vi "JSON Config Update Test Cases.vi"() -> ()   [LabVIEW 2021]
uses:
  CIFUtilities/CIFOutOfBand/CIFOutOfBand.lvclass/CIFOutOfBand.ctl
  CIFTemplateCoreOOB/OOB_Rx/Private/Command Settings.vi
  CIFUtilities/CIFOutOfBand/Accessors/Write Local OOB Data.vi
  CIFUtilities/CIFOutOfBand/Accessors/Read Local OOB Data.vi
  CIFUtilities/CIFOutOfBand/Read OOB DVR.vi
  CIFTemplateCoreOOB/OOB_Rx/Private/Read Payload.vi
  CIFUtilities/CIFOutOfBand/Write OOB DVR.vi
  CIFUtilities/CIFOutOfBand/Utilities/Command to Bitwise Command.vi
  CIFTemplateCoreOOB/OOB_Rx/CIFTemplateCoreOOB_Rx.lvclass
  D:/dev/CIF-Core-LabVIEW/src/CIFUtilities/CIFOutOfBand/CIFOutOfBand.lvclass
  CIFUtilities/CIFOutOfBand/Init OOB.vi
  <vilib>/addons/_JKI.lib/Serialization/JSON/Library/Unflatten From JSON String.vi
  <vilib>/addons/_JKI.lib/Serialization/JSON/JKI JSON Serialization.lvlib
  CIFUtilities/CIFOutOfBand/CIFOutOfBand.lvclass
panel:
  out "pass":bool
  out "error out":errorcluster
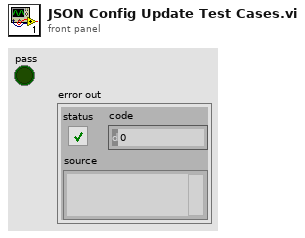
[diagram p1: front panel]
types:
  T1 = cluster{"Numeric":dbl, "String":string, "Boolean":bool}[]
  T2 = cluster{"Numeric":dbl, "Array":cluster{"Numeric":dbl, "String":string, "Boolean":bool}[], "string":string, "Null array":u8[]}
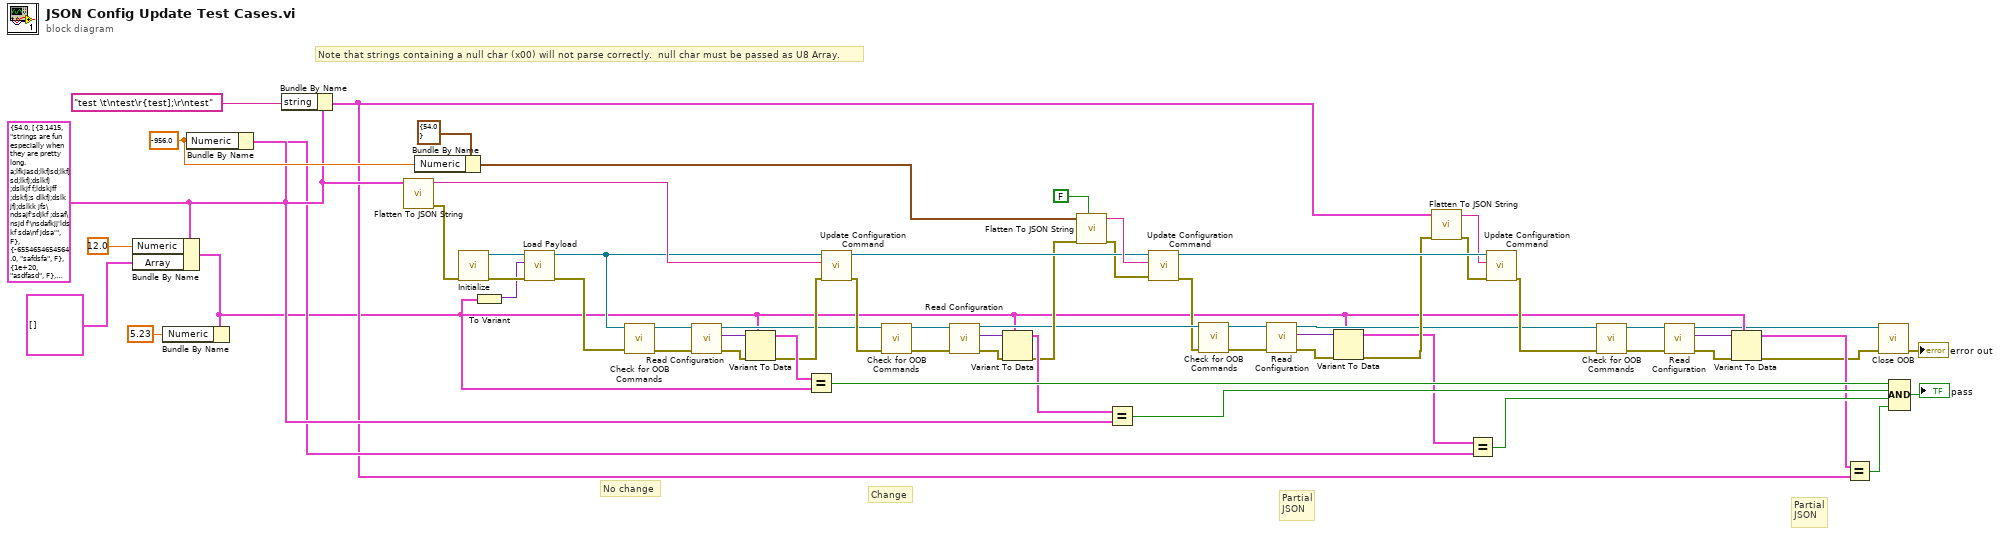
[diagram p0: block diagram]
diagram:
  w53 = -956.0 ("Numeric")
  w46 = T2 {"Numeric"=54.0, "Array"=[{"Numeric"=3.1415, "String"="strings are fun especially when they are pretty long. a;lfkjasd;lkfjsd;lkfjsd;lkfj;dslkfj ;dslkjf f;ldskjff ;dskfj;s dlkfj;dslk jfj;dslkk jfs\ndsajf'sdjkf ;dsaf\nsjd f'\nsdafkjj'lds kf sda\nf jdsa'", "Boolean"=FALSE}, {"Numeric"=-6554654654564.0, "String"="safdsfa", "Boolean"=FALSE}, {"Numeric"=1e+20, "String"="asdfasd", "Boolean"=FALSE}, {"Numeric"=2.0, "String"="afd", "Boolean"=TRUE}, {"Numeric"=12.34, "String"="data", "Boolean"=FALSE}], "string"="strings", "Null array"=[0]} ("Test Config")
  # "Note that strings containing a null char (x00) will not parse correctly.  null char must be passed as U8 Array."
  # "Partial\nJSON"
  # "Partial\nJSON"
  # "Change"
  # "No change"
  n1 = Bundle By Name(cluster=w46, "Numeric"=12.0, "Array"=T1 []) -> (w4:T2)
  n2 = Bundle By Name(cluster=w4, "Numeric"=5.23) -> ()  [unwired: 1 out]
  n3 = Bundle By Name(cluster=w46, "Numeric"=w53) -> (w45:T2)
  n4 = Bundle By Name(cluster=w46, "string"="test \t\ntest\r{test];\r\ntest" ("concatenated string")) -> (w41:T2)
  n5 = call <vilib>:"Flatten To JSON String.vi"("Variant"=w46) -> ("error out"=w58:errorcluster, "JSON String"=w60:string)  [unwired: 9 in]
  n6 = Bundle By Name(cluster=cluster{"Numeric":dbl} {"Numeric"=54.0} ("Test Config"), "Numeric"=w53) -> (w52:cluster{"Numeric":dbl})
  n7 = call "Initialize.vi"("error in"=w58) -> ("error out"=w37:errorcluster, "CoreOOB_Rx out"=w38:refnum<class "CIFTemplateCoreOOB_Rx.lvclass">)  [unwired: 9 in]
  n8 = To Variant(anything=w4) -> (Variant=w28:variant)
  n9 = call "Load Payload.vi"("error in (no error)"=w37, "Configuration Payload"=w28, "CoreOOB_Rx in"=w38) -> ("error out"=w36:errorcluster, "CoreOOB_Rx out"=w35:refnum<class "CIFTemplateCoreOOB_Rx.lvclass">)  [unwired: 7 in]
  n10 = call "Check for OOB Commands.vi"("error in (no error)"=w36, "CoreOOB_Rx in"=w35) -> ("error out"=w32:errorcluster, "CoreOOB_Rx out"=w33:refnum<class "CIFTemplateCoreOOB_Rx.lvclass">)  [unwired: 6 in, 2 out]
  n11 = call "Read Configuration.vi"("error in"=w32, "CoreOOB_Rx in"=w33) -> ("error out"=w30:errorcluster, "Configuration Data"=w31:variant, "CoreOOB_Rx out"=w21:refnum<class "CIFTemplateCoreOOB_Rx.lvclass">)  [unwired: 7 in]
  n12 = Variant To Data(error in=w30, type=w4, Variant=w31) -> (data=w29:T2, error out=w27:errorcluster)
  n13 = Equal?(x=w29, y=w4) -> (x = y?=w50:bool)
  n14 = call "Update Configuration Command.vi"("error in"=w27, "Config JSON"=w60, "CoreOOB_Rx in"=w35) -> ("error out"=w22:errorcluster, "CoreOOB_Rx out"=w55:refnum<class "CIFTemplateCoreOOB_Rx.lvclass">)  [unwired: 7 in]
  n15 = call "Check for OOB Commands.vi"("error in (no error)"=w22, "CoreOOB_Rx in"=w21) -> ("error out"=w24:errorcluster, "CoreOOB_Rx out"=w23:refnum<class "CIFTemplateCoreOOB_Rx.lvclass">)  [unwired: 6 in, 2 out]
  n16 = call "Read Configuration.vi"("error in"=w24, "CoreOOB_Rx in"=w23) -> ("error out"=w26:errorcluster, "Configuration Data"=w25:variant, "CoreOOB_Rx out"=w15:refnum<class "CIFTemplateCoreOOB_Rx.lvclass">)  [unwired: 7 in]
  n17 = Variant To Data(error in=w26, type=w4, Variant=w25) -> (data=w20:T2, error out=w19:errorcluster)
  n18 = call <vilib>:"Flatten To JSON String.vi"("Multiline (T)"=FALSE, "error in (no error)"=w19, "Variant"=w52) -> ("error out"=w51:errorcluster, "JSON String"=w56:string)  [unwired: 7 in]
  n19 = Equal?(x=w20, y=w46) -> (x = y?=w49:bool)
  n20 = call "Update Configuration Command.vi"("error in"=w51, "Config JSON"=w56, "CoreOOB_Rx in"=w55) -> ("error out"=w13:errorcluster, "CoreOOB_Rx out"=w44:refnum<class "CIFTemplateCoreOOB_Rx.lvclass">)  [unwired: 7 in]
  n21 = call "Check for OOB Commands.vi"("error in (no error)"=w13, "CoreOOB_Rx in"=w15) -> ("error out"=w18:errorcluster, "CoreOOB_Rx out"=w14:refnum<class "CIFTemplateCoreOOB_Rx.lvclass">)  [unwired: 6 in, 2 out]
  n22 = call "Read Configuration.vi"("error in"=w18, "CoreOOB_Rx in"=w14) -> ("error out"=w16:errorcluster, "Configuration Data"=w17:variant, "CoreOOB_Rx out"=w5:refnum<class "CIFTemplateCoreOOB_Rx.lvclass">)  [unwired: 7 in]
  n23 = Variant To Data(error in=w16, type=w4, Variant=w17) -> (data=w11:T2, error out=w12:errorcluster)
  n24 = call <vilib>:"Flatten To JSON String.vi"("error in (no error)"=w12, "Variant"=w41) -> ("error out"=w43:errorcluster, "JSON String"=w42:string)  [unwired: 8 in]
  n25 = Equal?(x=w11, y=w45) -> (x = y?=w48:bool)
  n26 = call "Update Configuration Command.vi"("error in"=w43, "Config JSON"=w42, "CoreOOB_Rx in"=w44) -> ("error out"=w6:errorcluster)  [unwired: 7 in, 1 out]
  n27 = call "Check for OOB Commands.vi"("error in (no error)"=w6, "CoreOOB_Rx in"=w5) -> ("error out"=w7:errorcluster, "CoreOOB_Rx out"=w10:refnum<class "CIFTemplateCoreOOB_Rx.lvclass">)  [unwired: 6 in, 2 out]
  n28 = call "Read Configuration.vi"("error in"=w7, "CoreOOB_Rx in"=w10) -> ("error out"=w9:errorcluster, "Configuration Data"=w8:variant, "CoreOOB_Rx out"=w2:refnum<class "CIFTemplateCoreOOB_Rx.lvclass">)  [unwired: 7 in]
  n29 = Variant To Data(error in=w9, type=w4, Variant=w8) -> (data=w3:T2, error out=w1:errorcluster)
  n30 = Equal?(x=w3, y=w41) -> (x = y?=w40:bool)
  n31 = call "Close OOB.vi"("error in"=w1, "OOB in"=w2) -> ("error out"=→"error out":errorcluster)  [unwired: 9 in]
  n32 = Compound Arithmetic op=AND(w50, w49, w48, w40) -> (→"pass":bool)
